vi "Prepare receive message (SubVI).vi"(5 "Connection in":refnum<class "Connection.lvclass">, 6 "error in (no error)":errorcluster, 7 "binding key":string[](array[string])=["broadcast.#"], 8 "exchange name":u16(ring) items=["requests", "alerts"], 9 "queue \nname":string) -> (0 "error out":errorcluster, 1 "Exchange.lvclass":refnum<class "Exchange.lvclass">, 2 "Queue out":refnum<class "Queue.lvclass">, 3 "Channel out":refnum<class "Channel.lvclass">, 4 "Connection out":refnum<class "Connection.lvclass">)   [LabVIEW 2016]
uses:
  <vilib>/Distrio/LabbitMQ/Connection/Connection.lvclass
  <vilib>/Distrio/LabbitMQ/Queue/Queue.lvclass
  <vilib>/Distrio/LabbitMQ/Exchange/Exchange.lvclass
  <vilib>/Distrio/LabbitMQ/Channel/Channel.lvclass
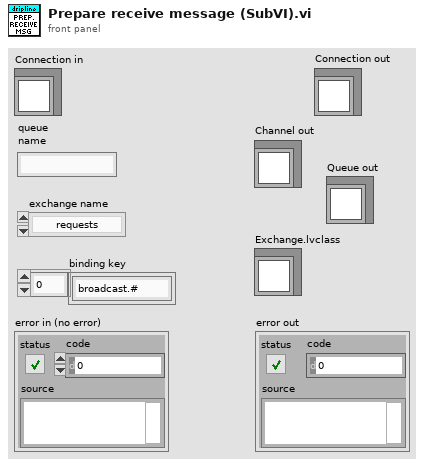
[diagram p1: front panel]
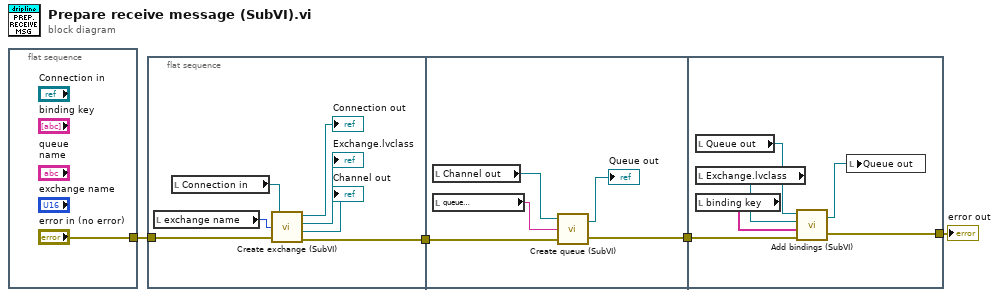
[diagram p0: block diagram]
diagram:
  n1 = flat-sequence {
    tunnel: ["error in (no error)"] -> w4
    frame #0 {
    }
  }
  n2 = flat-sequence {
    tunnel: w4 -> [w12]
    tunnel: [w11] -> w3
    tunnel: w3 -> [w17]
    tunnel: [w16] -> w2
    tunnel: w2 -> [w23]
    tunnel: [w22] -> w1
    frame #0 {
      n3 = local read "exchange name"() -> (w9:u16)
      n4 = local read "Connection in"() -> (w10:refnum<class "Connection.lvclass">)
      n5 = call "Create exchange (SubVI).vi"("Connection in"=w10, "exchange name"=w9, "error in (no error)"=w12) -> ("Connection out"=→"Connection out":refnum<class "Connection.lvclass">, "Exchange.lvclass"=→"Exchange.lvclass":refnum<class "Exchange.lvclass">, "Channel out"=→"Channel out":refnum<class "Channel.lvclass">, "error out"=w11:errorcluster)
    }
    frame #1 {
      n6 = local read "Channel out"() -> (w15:refnum<class "Channel.lvclass">)
      n7 = local read "queue \nname"() -> (w14:string)
      n8 = call "Create queue (SubVI).vi"("error in (no error)"=w17, "queue"=w14, "Channel in"=w15) -> ("error out"=w16:errorcluster, "Queue out"=→"Queue out":refnum<class "Queue.lvclass">)
    }
    frame #2 {
      n9 = local read "Queue out"() -> (w21:refnum<class "Queue.lvclass">)
      n10 = local read "Exchange.lvclass"() -> (w20:refnum<class "Exchange.lvclass">)
      n11 = local read "binding key"() -> (w19:string[])
      n12 = call "Add bindings (SubVI).vi"("error in (no error)"=w23, "binding key"=w19, "Exchange.lvclass"=w20, "Queue in"=w21) -> ("error out"=w22:errorcluster, "Queue out"=w18:refnum<class "Queue.lvclass">)
      n13 = local write "Queue out"(w18) -> ()
    }
  }
  "error out" <- w1
